vi "ber.vi"(8 "Key Bit Sequence":u32[](array[numeric]), 11 "Recovered Bit Sequence":u32[](array[numeric])) -> (3 "BER":dbl)   [LabVIEW 2012]
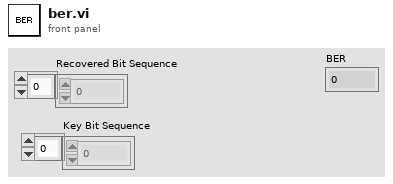
[diagram p1: front panel]
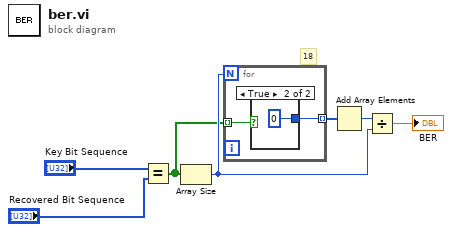
[diagram p0: block diagram]
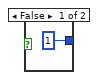
[diagram p2: hidden frame]
diagram:
  # "18"
  n1 = Equal?(x="Key Bit Sequence", y="Recovered Bit Sequence") -> (x = y?=w4:bool[])
  n2 = Array Size(array=w4) -> (size(s)=w5:i32)
  n3 = for {
    N: w5 -> [_]
    tunnel: [w9] -> w7 mode=indexing
    tunnel: w4 -> [w8] mode=indexing
    n4 = case shown="True" w8 {
      tunnel: [1 0] -> w9
      frame False {
      }
      frame True {
      }
    }
  }
  n5 = Add Array Elements(numeric array=w7) -> (sum=w6:i32)
  n6 = Divide(x=w6, y=w5) -> (x/y=→"BER":dbl)
